vi "TSM DMM Configure Settings.vi"(0 "DMM TSM In":T1, 5 "Function":T2, 7 "Range":dbl=10.0, 9 "Resolution in Digits":T3=7.5 items=["3 1/2"=3.5, "4 1/2"=4.5, "5 1/2"=5.5, "6 1/2"=6.5, "7 1/2"=7.5], 11 "error in":errorcluster, 12 "Aperture Time (s)":dbl=0.01666 format="%#_13p") -> (4 "DMM TSM Out":T1, 15 "error out":errorcluster)   [LabVIEW 2019]
doc: "Use this VI to configure the NI-DMM instruments in the pin map associated with the test program."
uses:
  <instrlib>/niDMM/nidmm.llb/niDMM Resolution in Digits.ctl
  <instrlib>/niDMM/nidmm.llb/niDMM Function.ctl
  Pin Map/TSM DMM.ctl
  <vilib>/NI_TestStand_SemiconductorModule/NI_TestStand_Semiconductor_Module.lvlibp/PinMap/PinQueryContext/MultiplePinMultipleSessionQueryContext/MultiplePinMultipleSessionQueryContext.lvclass
  <instrlib>/niDMM/nidmm.llb/niDMM Configure Measurement Digits.vi
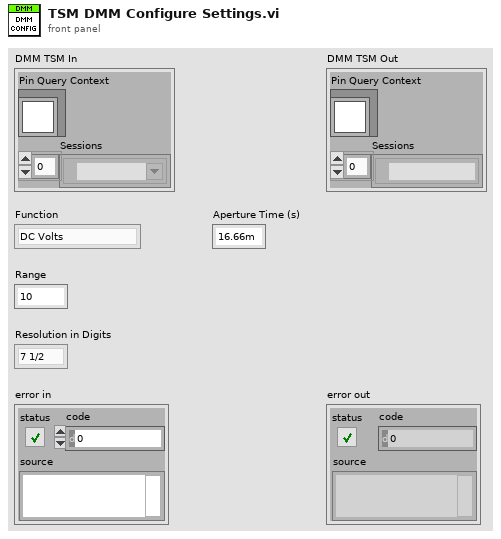
[diagram p1: front panel]
types:
  T1 = typedef "TSM DMM.ctl" = cluster{"Pin Query Context":refnum<class "MultiplePinMultipleSessionQueryContext.lvclass">, "Sessions":refnum<k15>[]}
  T2 = typedef "niDMM Function.ctl" = enum16{"DC Volts", "AC Volts", "DC Current", "AC Current", "2-wire Resistance", "4-wire Resistance", "Diode", "Frequency", "Period", "AC Volts DC Coupled", "Capacitance", "Inductance", "Temperature"}
  T3 = typedef "niDMM Resolution in Digits.ctl" = dbl
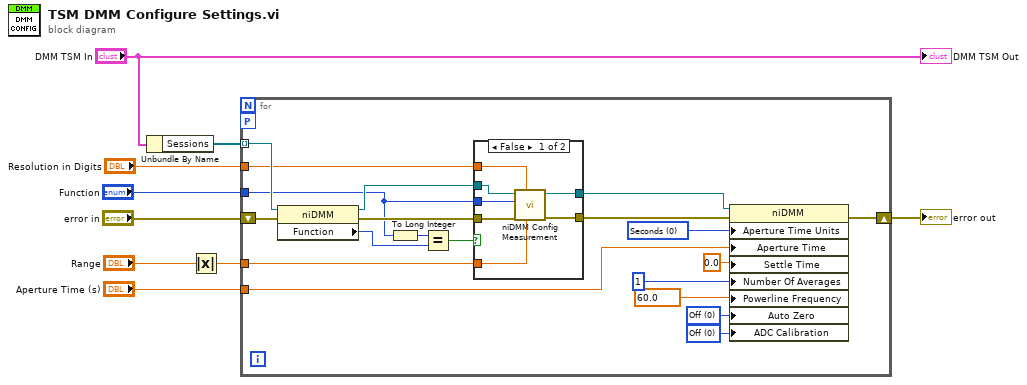
[diagram p0: block diagram]
diagram:
  n1 = Unbundle By Name("DMM TSM In") -> ("Sessions"=w2:refnum<k15>[])
  n2 = Absolute Value(x="Range") -> (abs(x)=w7:dbl)
  n3 = for {
    tunnel: "Resolution in Digits" -> [w13]
    tunnel: w7 -> [w29]
    tunnel: "Aperture Time (s)" -> [w25]
    tunnel: "Function" -> [w14]
    tunnel: w2 -> [w18] mode=indexing
    shift-right: [w19] -> w4
    shift-left: "error in" -> [w17]
    workers-P: _ -> [_]
    w10 = 0 items=["Auto"=-1, "Off"=0, "On"=1] ("Configuration:Measurement Options:ADC Calibration")
    w11 = 0 items=["Auto"=-1, "Off"=0, "On"=1, "Once"=2] ("Configuration:Measurement Options:Auto Zero")
    w23 = 60.0 items=["50 Hz"=50.0, "60 Hz"=60.0] ("Configuration:Measurement Options:Powerline Frequency")
    w24 = 0 items=["Seconds", "Power Line Cycles"] ("Configuration:Advanced:Aperture Time Units")
    n4 = property class="niDMM"(reference=w18, error in=w17) -> (reference out=w20:refnum<k15>, error out=w22:errorcluster, "Function"=w16:i32)
    n5 = To Long Integer(number=w14) -> (32bit integer=w15:i32)
    n6 = Equal?(x=w15, y=w16) -> (x = y?=w21:bool)
    n7 = case shown="False" w21 {
      tunnel: w13 -> [w36 _]
      tunnel: w29 -> [w35 _]
      tunnel: [w34 w38] -> w28
      tunnel: [w33 w37] -> w27
      tunnel: w22 -> [w32 w38]
      tunnel: w14 -> [w31 _]
      tunnel: w20 -> [w30 w37]
      frame False {
        n8 = call-poly <instrlib>:"niDMM Config Measurement.vi"("Range"=w35, "Resolution in Digits"=w36, "error in (no error)"=w32, "Function"=w31, "instrument handle"=w30) -> ("error out"=w34:errorcluster, "instrument handle out"=w33:refnum<k15>)  [unwired: 5 in]
      }
      frame True {
      }
    }
    n9 = property class="niDMM"(reference=w27, error in=w28, "Aperture Time Units"=w24, "Aperture Time"=w25, "Settle Time"=0.0 ("Configuration:Advanced:Settle Time"), "Number Of Averages"=1 ("Configuration:Advanced:Number Of Averages"), "Powerline Frequency"=w23, "Auto Zero"=w11, "ADC Calibration"=w10) -> (error out=w19:errorcluster)  [unwired: 1 out]
  }
  "error out" <- w4
  "DMM TSM Out" <- "DMM TSM In"
